vi "Uint8 Create.vi"(8 "error in (no error)":errorcluster, 11 "U8 in":u8) -> (0 "error out":errorcluster, 3 "Uint8 DVR out":refnum<data-value>)   [LabVIEW 2012, in "MDSplus.lvlib"]
uses:
  <vilib>/MDSplus/Library/MDSplus.lvlib
  <vilib>/MDSplus/Classes/Data_Class/Scalar_Class/Uint8_Class/Uint8.lvclass
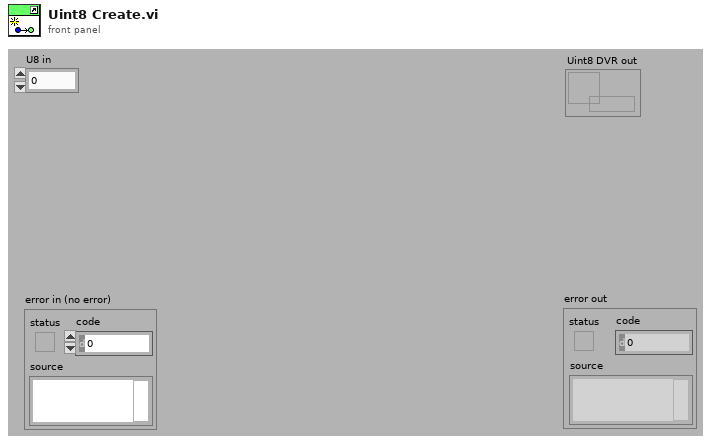
[diagram p1: front panel]
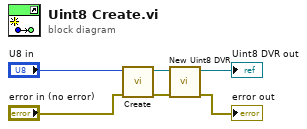
[diagram p0: block diagram]
diagram:
  n1 = call <vilib>:"Create.vi"("error in (no error)"="error in (no error)", "U8 in"="U8 in") -> ("error out"=w3:errorcluster, "Uint8 out"=w4:refnum<class "Uint8.lvclass">)  [unwired: 8 in]
  n2 = call <vilib>:"New Uint8 DVR.vi"("error in (no error)"=w3, "Uint8 in"=w4) -> ("error out"=→"error out":errorcluster, "Uint8 DVR out"=→"Uint8 DVR out":refnum<data-value>)  [unwired: 8 in]
